vi "数据发送组合-20200825 (子VI).vi"(10 "枚举":T2(ring), 11 "插值后的数组元素":T1) -> (3 "字符串":string)   [LabVIEW 2016, in "数据传输系统-02.lvlib"]
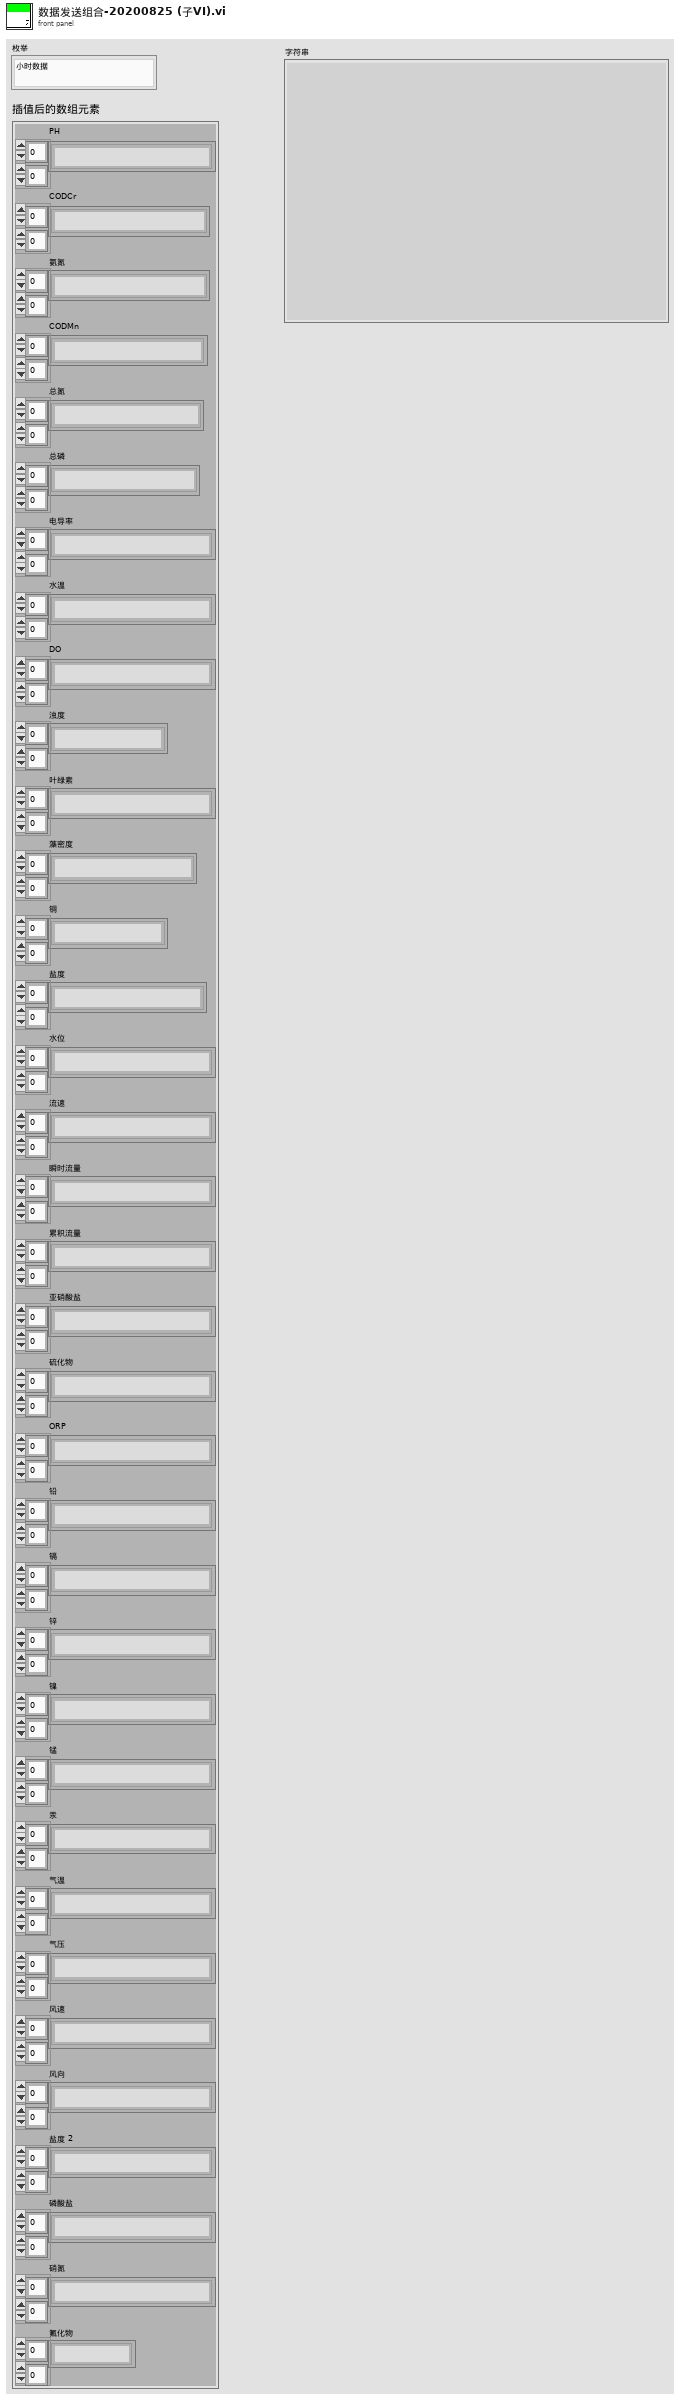
[diagram p1: front panel]
types:
  T1 = cluster{"PH":string[][], "CODCr":string[][], "氨氮":string[][], "CODMn":string[][], "总氮":string[][], "总磷":string[][], "电导率":string[][], "水温":string[][], "DO":string[][], "浊度":string[][], "叶绿素":string[][], "藻密度":string[][], "铜":string[][], "盐度":string[][], "水位":string[][], "流速":string[][], "瞬时流量":string[][], "累积流量":string[][], "亚硝酸盐":string[][], "硫化物":string[][], "ORP":string[][], "铅":string[][], "镉":string[][], "锌":string[][], "镍":string[][], "锰":string[][], "汞":string[][], "气温":string[][], "气压":string[][], "风速":string[][], "风向":string[][], "盐度 2":string[][], "磷酸盐":string[][], "硝氮":string[][], "氟化物":string[][]}
  T2 = enum16{"小时数据", "实时数据", "平行样测试", "集成干预测试", "加标回收测试", "核查数据", "空白零点跨度数据", "提取小时数据", "提取实时数据", "操作日志", "仪器参数", "3090仪器参数", "提取仪器参数", "报警信息"}
  T3 = cluster{"CODMn":dbl, "CODCr":dbl, "DO":dbl, "铜":dbl, "PH":dbl, "氨氮":dbl, "比电导率":dbl, "水温":dbl, "COD":dbl, "浊度":dbl, "总氮":dbl, "总磷":dbl, "叶绿素a":dbl, "藻密度":dbl, "水位":dbl, "流速":dbl, "瞬时流量":dbl, "累积流量":dbl, "亚硝酸盐":dbl, "硫化物":dbl, "ORP":dbl, "铅":dbl, "镉":dbl, "锌":dbl, "镍":dbl, "锰":dbl, "汞":dbl, "气温":dbl, "气压":dbl, "风速":dbl, "风向":dbl, "盐度":dbl, "磷酸盐":dbl, "硝氮":dbl, "氟化物":dbl}
  T4 = cluster{"CODMn":string, "CODCr":string, "DO":string, "铜":string, "PH":string, "氨氮":string, "比电导率":string, "水温":string, "COD":string, "浊度":string, "总氮":string, "总磷":string, "叶绿素a":string, "藻密度":string, "水位":string, "流速":string, "瞬时流量":string, "累积流量":string, "亚硝酸盐":string, "硫化物":string, "ORP":string, "铅":string, "镉":string, "锌":string, "镍":string, "锰":string, "汞":string, "气温":string, "气压":string, "风速":string, "风向":string, "盐度":string, "磷酸盐":string, "硝氮":string, "氟化物":string}
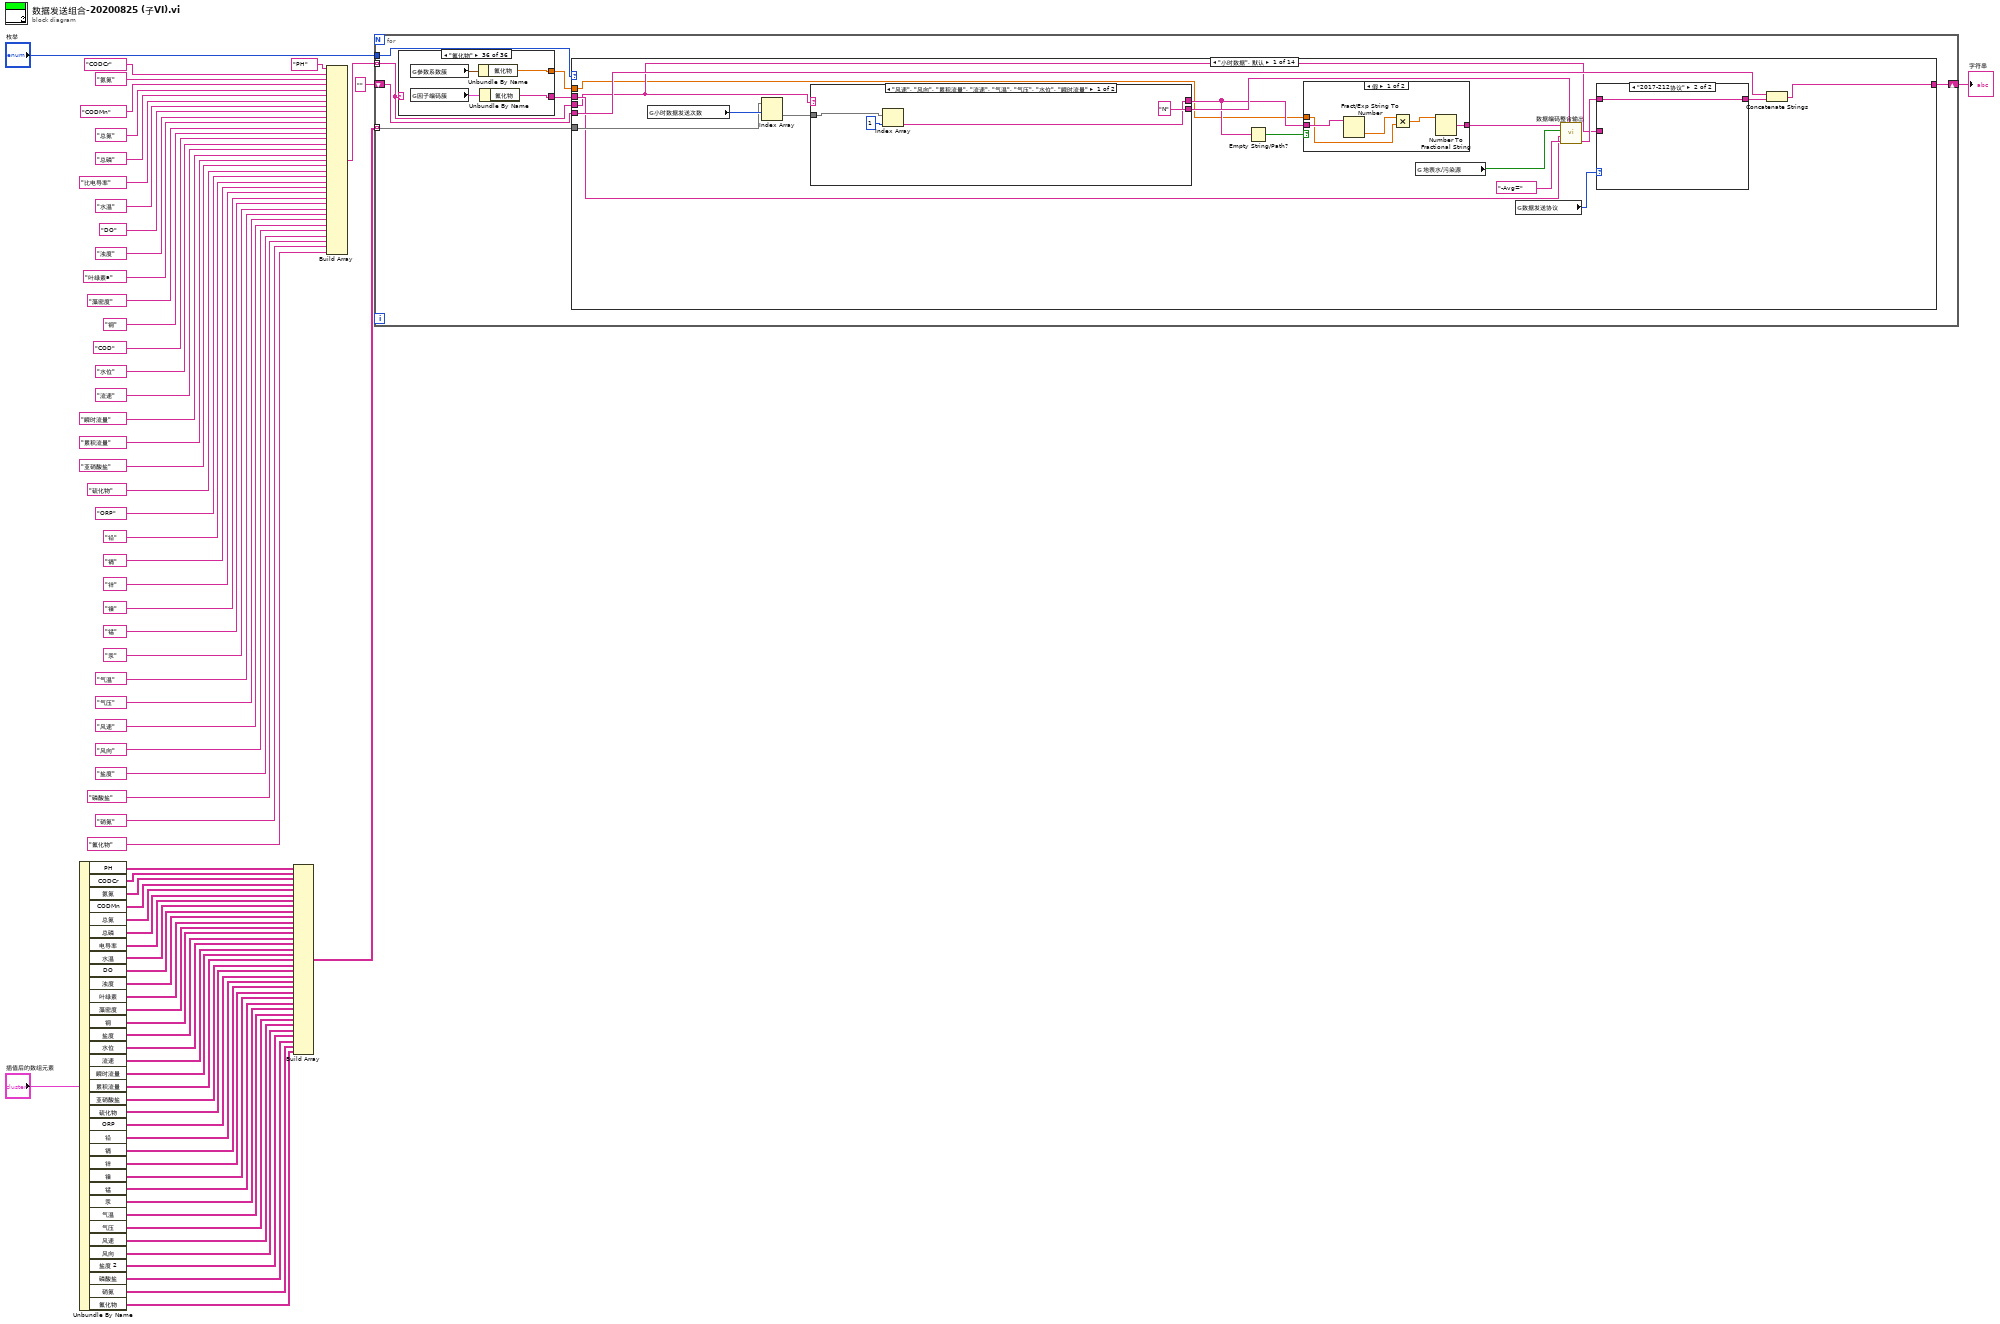
[diagram p0: block diagram]
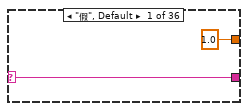
[diagram p2: hidden frame]
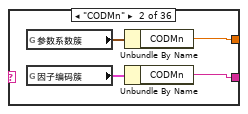
[diagram p3: hidden frame]
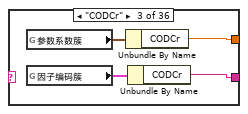
[diagram p4: hidden frame]
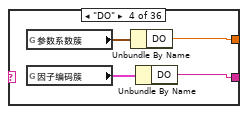
[diagram p5: hidden frame]
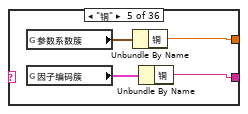
[diagram p6: hidden frame]
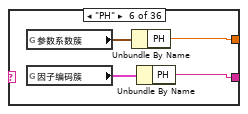
[diagram p7: hidden frame]
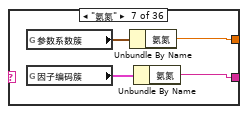
[diagram p8: hidden frame]
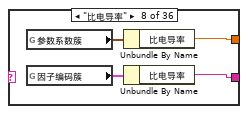
[diagram p9: hidden frame]
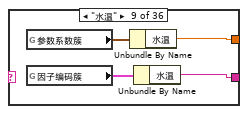
[diagram p10: hidden frame]
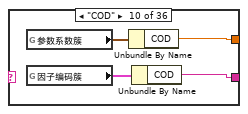
[diagram p11: hidden frame]
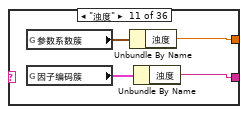
[diagram p12: hidden frame]
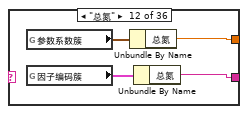
[diagram p13: hidden frame]
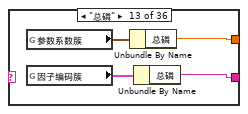
[diagram p14: hidden frame]
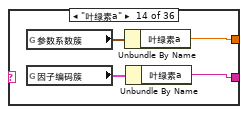
[diagram p15: hidden frame]
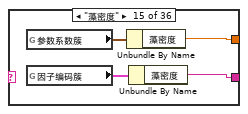
[diagram p16: hidden frame]
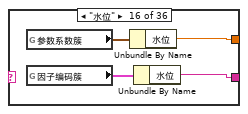
[diagram p17: hidden frame]
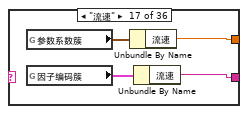
[diagram p18: hidden frame]
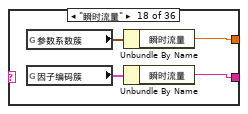
[diagram p19: hidden frame]
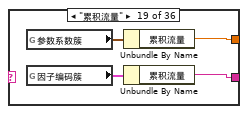
[diagram p20: hidden frame]
diagram:
  n1 = Unbundle By Name("插值后的数组元素") -> ("PH"=w76:string[][], "CODCr"=w75:string[][], "氨氮"=w74:string[][], "CODMn"=w73:string[][], "总氮"=w72:string[][], "总磷"=w71:string[][], "电导率"=w70:string[][], "水温"=w69:string[][], "DO"=w68:string[][], "浊度"=w67:string[][], "叶绿素"=w66:string[][], "藻密度"=w65:string[][], "铜"=w64:string[][], "盐度"=w63:string[][], "水位"=w62:string[][], "流速"=w61:string[][], "瞬时流量"=w60:string[][], "累积流量"=w59:string[][], "亚硝酸盐"=w58:string[][], "硫化物"=w57:string[][], "ORP"=w56:string[][], "铅"=w55:string[][], "镉"=w54:string[][], "锌"=w53:string[][], "镍"=w52:string[][], "锰"=w51:string[][], "汞"=w50:string[][], "气温"=w14:string[][], "气压"=w15:string[][], "风速"=w16:string[][], "风向"=w17:string[][], "盐度 2"=w8:string[][], "磷酸盐"=w7:string[][], "硝氮"=w6:string[][], "氟化物"=w2:string[][])
  n2 = Build Array(w76, w75, w74, w73, w72, w71, w70, w69, w68, w67, w66, w65, w64, w63, w62, w61, w60, w59, w58, w57, w56, w55, w54, w53, w52, w51, w50, w14, w15, w16, w17, w8, w7, w6, w2) -> (w49:string[][][])
  n3 = Build Array("PH" ("污染物编码"), "CODCr" ("污染物编码"), "氨氮" ("污染物编码"), "CODMn" ("污染物编码"), "总氮" ("污染物编码"), "总磷" ("污染物编码"), "比电导率" ("污染物编码"), "水温" ("污染物编码"), "DO" ("污染物编码"), "浊度" ("污染物编码"), "叶绿素a" ("污染物编码"), "藻密度" ("污染物编码"), "铜" ("污染物编码"), "COD" ("污染物编码"), "水位" ("污染物编码"), "流速" ("污染物编码"), "瞬时流量" ("污染物编码"), "累积流量" ("污染物编码"), "亚硝酸盐" ("污染物编码"), "硫化物" ("污染物编码"), "ORP" ("污染物编码"), "铅" ("污染物编码"), "镉" ("污染物编码"), "锌" ("污染物编码"), "镍" ("污染物编码"), "锰" ("污染物编码"), "汞" ("污染物编码"), "气温" ("污染物编码"), "气压" ("污染物编码"), "风速" ("污染物编码"), "风向" ("污染物编码"), "盐度" ("污染物编码"), "磷酸盐" ("污染物编码"), "硝氮" ("污染物编码"), "氟化物" ("污染物编码")) -> (w21:string[])
  n4 = for {
    tunnel: w49 -> [w83] mode=indexing
    tunnel: w21 -> [w78] mode=indexing
    shift-right: [w82] -> w19
    shift-left: "" -> [w81]
    tunnel: "枚举" -> [w80]
    n5 = case shown="\"氟化物\"" w78 {
      selector: w78 -> [w85 _ _ _ _ _ _ _ _ _ _ _ _ _ _ _ _ _ _ _ _ _ _ _ _ _ _ _ _ _ _ _ _ _ _ _]
      tunnel: [w85 w88 w92 w96 w100 w104 w108 w112 w116 w120 w124 w128 w132 w136 w140 w144 w148 w152 w156 w160 w164 w168 w172 w176 w180 w184 w188 w192 w196 w200 w204 w208 w212 w216 w220 w224] -> w79
      tunnel: [1.0 ("风向") w86 w90 w94 w98 w102 w106 w110 w114 w118 w122 w126 w130 w134 w138 w142 w146 w150 w154 w158 w162 w166 w170 w174 w178 w182 w186 w190 w194 w198 w202 w206 w210 w214 w218 w222] -> w77
      frame "假", Default {
      }
      frame "CODMn" {
        n6 = global read "断电保存全局.vi" "参数系数簇"() -> (w87:T3)
        n7 = global read "断电保存全局.vi" "因子编码簇"() -> (w89:T4)
        n8 = Unbundle By Name(w87) -> ("CODMn"=w86:dbl)
        n9 = Unbundle By Name(w89) -> ("CODMn"=w88:string)
      }
      frame "CODCr" {
        n10 = global read "断电保存全局.vi" "参数系数簇"() -> (w91:T3)
        n11 = global read "断电保存全局.vi" "因子编码簇"() -> (w93:T4)
        n12 = Unbundle By Name(w91) -> ("CODCr"=w90:dbl)
        n13 = Unbundle By Name(w93) -> ("CODCr"=w92:string)
      }
      frame "DO" {
        n14 = global read "断电保存全局.vi" "参数系数簇"() -> (w95:T3)
        n15 = global read "断电保存全局.vi" "因子编码簇"() -> (w97:T4)
        n16 = Unbundle By Name(w95) -> ("DO"=w94:dbl)
        n17 = Unbundle By Name(w97) -> ("DO"=w96:string)
      }
      frame "铜" {
        n18 = global read "断电保存全局.vi" "参数系数簇"() -> (w99:T3)
        n19 = global read "断电保存全局.vi" "因子编码簇"() -> (w101:T4)
        n20 = Unbundle By Name(w99) -> ("铜"=w98:dbl)
        n21 = Unbundle By Name(w101) -> ("铜"=w100:string)
      }
      frame "PH" {
        n22 = global read "断电保存全局.vi" "参数系数簇"() -> (w103:T3)
        n23 = global read "断电保存全局.vi" "因子编码簇"() -> (w105:T4)
        n24 = Unbundle By Name(w103) -> ("PH"=w102:dbl)
        n25 = Unbundle By Name(w105) -> ("PH"=w104:string)
      }
      frame "氨氮" {
        n26 = global read "断电保存全局.vi" "参数系数簇"() -> (w107:T3)
        n27 = global read "断电保存全局.vi" "因子编码簇"() -> (w109:T4)
        n28 = Unbundle By Name(w107) -> ("氨氮"=w106:dbl)
        n29 = Unbundle By Name(w109) -> ("氨氮"=w108:string)
      }
      frame "比电导率" {
        n30 = global read "断电保存全局.vi" "参数系数簇"() -> (w111:T3)
        n31 = global read "断电保存全局.vi" "因子编码簇"() -> (w113:T4)
        n32 = Unbundle By Name(w111) -> ("比电导率"=w110:dbl)
        n33 = Unbundle By Name(w113) -> ("比电导率"=w112:string)
      }
      frame "水温" {
        n34 = global read "断电保存全局.vi" "参数系数簇"() -> (w115:T3)
        n35 = global read "断电保存全局.vi" "因子编码簇"() -> (w117:T4)
        n36 = Unbundle By Name(w115) -> ("水温"=w114:dbl)
        n37 = Unbundle By Name(w117) -> ("水温"=w116:string)
      }
      frame "COD" {
        n38 = global read "断电保存全局.vi" "参数系数簇"() -> (w119:T3)
        n39 = global read "断电保存全局.vi" "因子编码簇"() -> (w121:T4)
        n40 = Unbundle By Name(w119) -> ("COD"=w118:dbl)
        n41 = Unbundle By Name(w121) -> ("COD"=w120:string)
      }
      frame "浊度" {
        n42 = global read "断电保存全局.vi" "参数系数簇"() -> (w123:T3)
        n43 = global read "断电保存全局.vi" "因子编码簇"() -> (w125:T4)
        n44 = Unbundle By Name(w123) -> ("浊度"=w122:dbl)
        n45 = Unbundle By Name(w125) -> ("浊度"=w124:string)
      }
      frame "总氮" {
        n46 = global read "断电保存全局.vi" "参数系数簇"() -> (w127:T3)
        n47 = global read "断电保存全局.vi" "因子编码簇"() -> (w129:T4)
        n48 = Unbundle By Name(w127) -> ("总氮"=w126:dbl)
        n49 = Unbundle By Name(w129) -> ("总氮"=w128:string)
      }
      frame "总磷" {
        n50 = global read "断电保存全局.vi" "参数系数簇"() -> (w131:T3)
        n51 = global read "断电保存全局.vi" "因子编码簇"() -> (w133:T4)
        n52 = Unbundle By Name(w131) -> ("总磷"=w130:dbl)
        n53 = Unbundle By Name(w133) -> ("总磷"=w132:string)
      }
      frame "叶绿素a" {
        n54 = global read "断电保存全局.vi" "参数系数簇"() -> (w135:T3)
        n55 = global read "断电保存全局.vi" "因子编码簇"() -> (w137:T4)
        n56 = Unbundle By Name(w135) -> ("叶绿素a"=w134:dbl)
        n57 = Unbundle By Name(w137) -> ("叶绿素a"=w136:string)
      }
      frame "藻密度" {
        n58 = global read "断电保存全局.vi" "参数系数簇"() -> (w139:T3)
        n59 = global read "断电保存全局.vi" "因子编码簇"() -> (w141:T4)
        n60 = Unbundle By Name(w139) -> ("藻密度"=w138:dbl)
        n61 = Unbundle By Name(w141) -> ("藻密度"=w140:string)
      }
      frame "水位" {
        n62 = global read "断电保存全局.vi" "参数系数簇"() -> (w143:T3)
        n63 = global read "断电保存全局.vi" "因子编码簇"() -> (w145:T4)
        n64 = Unbundle By Name(w143) -> ("水位"=w142:dbl)
        n65 = Unbundle By Name(w145) -> ("水位"=w144:string)
      }
      frame "流速" {
        n66 = global read "断电保存全局.vi" "参数系数簇"() -> (w147:T3)
        n67 = global read "断电保存全局.vi" "因子编码簇"() -> (w149:T4)
        n68 = Unbundle By Name(w147) -> ("流速"=w146:dbl)
        n69 = Unbundle By Name(w149) -> ("流速"=w148:string)
      }
      frame "瞬时流量" {
        n70 = global read "断电保存全局.vi" "参数系数簇"() -> (w151:T3)
        n71 = global read "断电保存全局.vi" "因子编码簇"() -> (w153:T4)
        n72 = Unbundle By Name(w151) -> ("瞬时流量"=w150:dbl)
        n73 = Unbundle By Name(w153) -> ("瞬时流量"=w152:string)
      }
      frame "累积流量" {
        n74 = global read "断电保存全局.vi" "参数系数簇"() -> (w155:T3)
        n75 = global read "断电保存全局.vi" "因子编码簇"() -> (w157:T4)
        n76 = Unbundle By Name(w155) -> ("累积流量"=w154:dbl)
        n77 = Unbundle By Name(w157) -> ("累积流量"=w156:string)
      }
      frame "亚硝酸盐" {
        n78 = global read "断电保存全局.vi" "参数系数簇"() -> (w159:T3)
        n79 = global read "断电保存全局.vi" "因子编码簇"() -> (w161:T4)
        n80 = Unbundle By Name(w159) -> ("亚硝酸盐"=w158:dbl)
        n81 = Unbundle By Name(w161) -> ("亚硝酸盐"=w160:string)
      }
      frame "硫化物" {
        n82 = global read "断电保存全局.vi" "参数系数簇"() -> (w163:T3)
        n83 = global read "断电保存全局.vi" "因子编码簇"() -> (w165:T4)
        n84 = Unbundle By Name(w163) -> ("硫化物"=w162:dbl)
        n85 = Unbundle By Name(w165) -> ("硫化物"=w164:string)
      }
      frame "ORP" {
        n86 = global read "断电保存全局.vi" "参数系数簇"() -> (w167:T3)
        n87 = global read "断电保存全局.vi" "因子编码簇"() -> (w169:T4)
        n88 = Unbundle By Name(w167) -> ("ORP"=w166:dbl)
        n89 = Unbundle By Name(w169) -> ("ORP"=w168:string)
      }
      frame "铅" {
        n90 = global read "断电保存全局.vi" "参数系数簇"() -> (w171:T3)
        n91 = global read "断电保存全局.vi" "因子编码簇"() -> (w173:T4)
        n92 = Unbundle By Name(w171) -> ("铅"=w170:dbl)
        n93 = Unbundle By Name(w173) -> ("铅"=w172:string)
      }
      frame "镉" {
        n94 = global read "断电保存全局.vi" "参数系数簇"() -> (w175:T3)
        n95 = global read "断电保存全局.vi" "因子编码簇"() -> (w177:T4)
        n96 = Unbundle By Name(w175) -> ("镉"=w174:dbl)
        n97 = Unbundle By Name(w177) -> ("镉"=w176:string)
      }
      frame "锌" {
        n98 = global read "断电保存全局.vi" "参数系数簇"() -> (w179:T3)
        n99 = global read "断电保存全局.vi" "因子编码簇"() -> (w181:T4)
        n100 = Unbundle By Name(w179) -> ("锌"=w178:dbl)
        n101 = Unbundle By Name(w181) -> ("锌"=w180:string)
      }
      frame "镍" {
        n102 = global read "断电保存全局.vi" "参数系数簇"() -> (w183:T3)
        n103 = global read "断电保存全局.vi" "因子编码簇"() -> (w185:T4)
        n104 = Unbundle By Name(w183) -> ("镍"=w182:dbl)
        n105 = Unbundle By Name(w185) -> ("镍"=w184:string)
      }
      frame "锰" {
        n106 = global read "断电保存全局.vi" "参数系数簇"() -> (w187:T3)
        n107 = global read "断电保存全局.vi" "因子编码簇"() -> (w189:T4)
        n108 = Unbundle By Name(w187) -> ("锰"=w186:dbl)
        n109 = Unbundle By Name(w189) -> ("锰"=w188:string)
      }
      frame "汞" {
        n110 = global read "断电保存全局.vi" "参数系数簇"() -> (w191:T3)
        n111 = global read "断电保存全局.vi" "因子编码簇"() -> (w193:T4)
        n112 = Unbundle By Name(w191) -> ("汞"=w190:dbl)
        n113 = Unbundle By Name(w193) -> ("汞"=w192:string)
      }
      frame "气温" {
        n114 = global read "断电保存全局.vi" "参数系数簇"() -> (w195:T3)
        n115 = global read "断电保存全局.vi" "因子编码簇"() -> (w197:T4)
        n116 = Unbundle By Name(w195) -> ("气温"=w194:dbl)
        n117 = Unbundle By Name(w197) -> ("气温"=w196:string)
      }
      frame "气压" {
        n118 = global read "断电保存全局.vi" "参数系数簇"() -> (w199:T3)
        n119 = global read "断电保存全局.vi" "因子编码簇"() -> (w201:T4)
        n120 = Unbundle By Name(w199) -> ("气压"=w198:dbl)
        n121 = Unbundle By Name(w201) -> ("气压"=w200:string)
      }
      frame "风速" {
        n122 = global read "断电保存全局.vi" "参数系数簇"() -> (w203:T3)
        n123 = global read "断电保存全局.vi" "因子编码簇"() -> (w205:T4)
        n124 = Unbundle By Name(w203) -> ("风速"=w202:dbl)
        n125 = Unbundle By Name(w205) -> ("风速"=w204:string)
      }
      frame "风向" {
        n126 = global read "断电保存全局.vi" "参数系数簇"() -> (w207:T3)
        n127 = global read "断电保存全局.vi" "因子编码簇"() -> (w209:T4)
        n128 = Unbundle By Name(w207) -> ("风向"=w206:dbl)
        n129 = Unbundle By Name(w209) -> ("风向"=w208:string)
      }
      frame "盐度" {
        n130 = global read "断电保存全局.vi" "参数系数簇"() -> (w211:T3)
        n131 = global read "断电保存全局.vi" "因子编码簇"() -> (w213:T4)
        n132 = Unbundle By Name(w211) -> ("盐度"=w210:dbl)
        n133 = Unbundle By Name(w213) -> ("盐度"=w212:string)
      }
      frame "磷酸盐" {
        n134 = global read "断电保存全局.vi" "参数系数簇"() -> (w215:T3)
        n135 = global read "断电保存全局.vi" "因子编码簇"() -> (w217:T4)
        n136 = Unbundle By Name(w215) -> ("磷酸盐"=w214:dbl)
        n137 = Unbundle By Name(w217) -> ("磷酸盐"=w216:string)
      }
      frame "硝氮" {
        n138 = global read "断电保存全局.vi" "参数系数簇"() -> (w219:T3)
        n139 = global read "断电保存全局.vi" "因子编码簇"() -> (w221:T4)
        n140 = Unbundle By Name(w219) -> ("硝氮"=w218:dbl)
        n141 = Unbundle By Name(w221) -> ("硝氮"=w220:string)
      }
      frame "氟化物" {
        n142 = global read "断电保存全局.vi" "参数系数簇"() -> (w223:T3)
        n143 = global read "断电保存全局.vi" "因子编码簇"() -> (w225:T4)
        n144 = Unbundle By Name(w223) -> ("氟化物"=w222:dbl)
        n145 = Unbundle By Name(w225) -> ("氟化物"=w224:string)
      }
    }
    n146 = case shown="\"小时数据\", 默认" w80 {
      tunnel: w83 -> [w238 w282 w313 w322 w376 w383 w393 w417 w439 w476 w494 w501 w511 w533]
      tunnel: w79 -> [w234 w275 w312 w323 w377 w382 w392 w411 w438 w464 w492 w499 w510 w536]
      tunnel: [w237 w279 w314 w320 w378 w379 w389 w408 w437 w471 w489 w498 w506 w521] -> w82
      tunnel: w81 -> [w236 w280 w316 w321 w373 w381 w390 w409 w440 w472 w490 w500 w507 w516]
      tunnel: w78 -> [w231 w274 _ w317 _ _ _ _ _ _ _ _ _ w531]
      tunnel: w77 -> [w228 w270 _ w318 _ _ _ w404 w433 _ _ _ _ _]
      frame "小时数据", Default {
        n147 = global read "全局 小时数据发送次数.vi" "小时数据发送次数"() -> (w242:i32)
        n148 = Index Array(array=w238, index (row)=w242) -> (element=w241:string[])  [unwired: 1 in]
        n149 = case shown="\"风速\", \"风向\", \"累积流量\", \"流速\", \"气温\", \"气压\", \"水位\", \"瞬时流量\"" w231 {
          tunnel: w241 -> [w252 w255]
          tunnel: [w249 w254] -> w229
          tunnel: ["N" ("字符串") w253] -> w239
          frame "风速", "风向", "累积流量", "流速", "气温", "气压", "水位", "瞬时流量" {
            n150 = Index Array(array=w252, index=1 ("索引")) -> (element=w249:string)
          }
          frame "", Default {
            n151 = Index Array(array=w255, index #1=2 ("索引"), index #2=3 ("索引"), index #3=5 ("索引")) -> (element #1=w258:string, element #2=w257:string, element #3=w253:string)
            n152 = case shown="\"N\", 默认" w258 {
              tunnel: [w261 ""] -> w254
              tunnel: w257 -> [w261 _]
              frame "N", Default {
              }
              frame "M" {
              }
            }
          }
        }
        n153 = Empty String/Path?(string/path=w229) -> (empty?=w230:bool)
        n154 = case shown="假" w230 {
          tunnel: w229 -> [w246 w248]
          tunnel: w228 -> [w245 _]
          tunnel: [w243 w248] -> w227
          frame False {
            n155 = Fract/Exp String To Number(string=w246) -> (number=w247:dbl)  [unwired: 3 in, 1 out]
            n156 = Multiply(x=w247, y=w245) -> (x*y=w244:dbl)
            n157 = Number To Fractional String(number=w244) -> (F-format string=w243:string)  [unwired: 3 in]
          }
          frame True {
            # "空"
          }
        }
        n158 = global read "断电保存全局.vi" "地表水/污染源"() -> (w226:bool)
        n159 = global read "断电保存全局.vi" "数据发送协议"() -> (w235:enum16{"2005-212协议", "2017-212协议"})
        n160 = call "数据编码整合输出.vi"("数据标识"=w239, "数据类型"="-Avg=", "污染物编码"=w234, "地表水/污染源"=w226, "数据值"=w227) -> ("编码输出"=w233:string)  [unwired: 6 in]
        n161 = case shown="\"2017-212协议\"" w235 {
          tunnel: w231 -> [w265 _]
          tunnel: w233 -> [w263 w268]
          tunnel: [w264 w268] -> w232
          frame "2005-212协议", Default {
            n162 = case shown="\"风速\", \"风向\", \"累积流量\", \"流速\", \"气温\", \"气压\", \"水位\"" w265 {
              tunnel: [w266 ""] -> w264
              tunnel: w263 -> [w266 _]
              frame "假", Default {
              }
              frame "风速", "风向", "累积流量", "流速", "气温", "气压", "水位" {
              }
            }
          }
          frame "2017-212协议" {
          }
        }
        n163 = Concatenate Strings(w236, w232) -> (w237:string)
      }
      frame "实时数据" {
        n164 = global read "全局 小时数据发送次数.vi" "小时数据发送次数"() -> (w283:i32)
        n165 = Index Array(array=w282, index (row)=w283) -> (element=w284:string[])  [unwired: 1 in]
        n166 = case shown="\"\", 默认" w274 {
          tunnel: w284 -> [w293 w297 w303]
          tunnel: [w292 w296 w302] -> w272
          tunnel: ["N" ("字符串") "N" ("字符串") w300] -> w281
          frame "累积流量", "流速", "水位", "瞬时流量" {
            n167 = Index Array(array=w293, index=1 ("索引")) -> (element=w292:string)
          }
          frame "风速", "风向", "气温", "气压" {
            n168 = Index Array(array=w297, index=1 ("索引")) -> (element=w296:string)
          }
          frame "", Default {
            n169 = Index Array(array=w303, index #1=3 ("索引"), index #2=5 ("索引")) -> (element #1=w302:string, element #2=w300:string)
          }
        }
        n170 = Empty String/Path?(string/path=w272) -> (empty?=w273:bool)
        n171 = case shown="假" w273 {
          tunnel: w272 -> [w289 w291]
          tunnel: w270 -> [w288 _]
          tunnel: [w286 w291] -> w271
          frame False {
            n172 = Fract/Exp String To Number(string=w289) -> (number=w290:dbl)  [unwired: 3 in, 1 out]
            n173 = Multiply(x=w290, y=w288) -> (x*y=w287:dbl)
            n174 = Number To Fractional String(number=w287) -> (F-format string=w286:string)  [unwired: 3 in]
          }
          frame True {
            # "空"
          }
        }
        n175 = global read "断电保存全局.vi" "数据发送协议"() -> (w278:enum16{"2005-212协议", "2017-212协议"})
        n176 = call "数据编码整合输出.vi"("数据标识"=w281, "数据类型"="-Rtd=", "污染物编码"=w275, "地表水/污染源"=FALSE, "数据值"=w271) -> ("编码输出"=w277:string)  [unwired: 6 in]
        n177 = case shown="\"2017-212协议\"" w278 {
          tunnel: w274 -> [w307 _]
          tunnel: w277 -> [w305 w310]
          tunnel: [w306 w310] -> w276
          frame "2005-212协议", Default {
            n178 = case shown="\"假\", 默认" w307 {
              tunnel: [w308 ""] -> w306
              tunnel: w305 -> [w308 _]
              frame "假", Default {
              }
              frame "风速", "风向", "累积流量", "流速", "气温", "气压", "水位" {
              }
            }
          }
          frame "2017-212协议" {
          }
        }
        n179 = Concatenate Strings(w280, w276) -> (w279:string)
      }
      frame "平行样测试" {
        n180 = global read "全局 小时数据发送次数.vi" "小时数据发送次数"() -> (w311:i32)
        n181 = call "平行样集成干预数据组合(子VI).vi"("污染物编码"=w312, "数据输入"=w313, "小时数据发送次数"=w311) -> ("输出组合"=w315:string)  [unwired: 8 in]
        n182 = Concatenate Strings(w316, w315) -> (w314:string)
      }
      frame "集成干预测试" {
        n183 = global read "断电保存全局.vi" "应用环境"() -> (w319:enum16{"STD", "GB212"})
        n184 = case shown="\"GB212\"" w319 {
          tunnel: w323 -> [w327 w333]
          tunnel: w322 -> [w326 w334]
          tunnel: w321 -> [w325 w335]
          tunnel: [w324 w330] -> w320
          tunnel: w318 -> [_ w332]
          tunnel: w317 -> [_ w331]
          frame "STD", Default {
            n185 = global read "全局 小时数据发送次数.vi" "小时数据发送次数"() -> (w328:i32)
            n186 = call "平行样集成干预数据组合(子VI).vi"("污染物编码"=w327, "数据输入"=w326, "小时数据发送次数"=w328) -> ("输出组合"=w329:string)  [unwired: 8 in]
            n187 = Concatenate Strings(w325, w329) -> (w324:string)
          }
          frame "GB212" {
            n188 = global read "全局 小时数据发送次数.vi" "小时数据发送次数"() -> (w346:i32)
            n189 = Index Array(array=w334, index (row)=w346) -> (element=w345:string[])  [unwired: 1 in]
            n190 = case shown="\"\", 默认" w331 {
              tunnel: w345 -> [w356 w359]
              tunnel: [w353 w358] -> w338
              tunnel: ["N" ("字符串") w357] -> w343
              frame "风速", "风向", "累积流量", "流速", "气温", "气压", "水位", "瞬时流量" {
                n191 = Index Array(array=w356, index=1 ("索引")) -> (element=w353:string)
              }
              frame "", Default {
                n192 = Index Array(array=w359, index #1=2 ("索引"), index #2=3 ("索引"), index #3=5 ("索引")) -> (element #1=w362:string, element #2=w361:string, element #3=w357:string)
                n193 = case shown="\"N\", 默认" w362 {
                  tunnel: [w365 ""] -> w358
                  tunnel: w361 -> [w365 _]
                  frame "N", Default {
                  }
                  frame "M" {
                  }
                }
              }
            }
            n194 = Empty String/Path?(string/path=w338) -> (empty?=w339:bool)
            n195 = case shown="假" w339 {
              tunnel: w338 -> [w350 w352]
              tunnel: w332 -> [w349 _]
              tunnel: [w347 w352] -> w337
              frame False {
                n196 = Fract/Exp String To Number(string=w350) -> (number=w351:dbl)  [unwired: 3 in, 1 out]
                n197 = Multiply(x=w351, y=w349) -> (x*y=w348:dbl)
                n198 = Number To Fractional String(number=w348) -> (F-format string=w347:string)  [unwired: 3 in]
              }
              frame True {
                # "空"
              }
            }
            n199 = global read "断电保存全局.vi" "地表水/污染源"() -> (w336:bool)
            n200 = global read "断电保存全局.vi" "数据发送协议"() -> (w342:enum16{"2005-212协议", "2017-212协议"})
            n201 = call "数据编码整合输出.vi"("数据标识"=w343, "数据类型"="-Avg=", "污染物编码"=w333, "地表水/污染源"=w336, "数据值"=w337) -> ("编码输出"=w341:string)  [unwired: 6 in]
            n202 = case shown="\"2017-212协议\"" w342 {
              tunnel: w331 -> [w369 _]
              tunnel: w341 -> [w367 w372]
              tunnel: [w368 w372] -> w340
              frame "2005-212协议", Default {
                n203 = case shown="\"假\", 默认" w369 {
                  tunnel: [w370 ""] -> w368
                  tunnel: w367 -> [w370 _]
                  frame "假", Default {
                  }
                  frame "风速", "风向", "累积流量", "流速", "气温", "气压", "水位" {
                  }
                }
              }
              frame "2017-212协议" {
              }
            }
            n204 = Concatenate Strings(w335, w340) -> (w330:string)
          }
        }
      }
      frame "加标回收测试" {
        n205 = global read "全局 小时数据发送次数.vi" "小时数据发送次数"() -> (w375:i32)
        n206 = call "加标回收数据组合 (子VI).vi"("小时数据发送次数"=w375, "数据"=w376, "污染物编码"=w377) -> ("组合输出"=w374:string)  [unwired: 7 in, 1 out]
        n207 = Concatenate Strings(w373, w374) -> (w378:string)
      }
      frame "核查数据" {
        n208 = global read "全局 小时数据发送次数.vi" "小时数据发送次数"() -> (w384:i32)
        n209 = call "标样核查数据组合(子VI).vi"("小时数据发送次数"=w384, "数据输入"=w383, "污染物编码"=w382) -> ("输出组合"=w380:string)  [unwired: 8 in]
        n210 = Concatenate Strings(w381, w380) -> (w379:string)
      }
      frame "空白零点跨度数据" {
        n211 = global read "全局 小时数据发送次数.vi" "小时数据发送次数"() -> (w395:i32)
        n212 = Index Array(array=w393, index (row)=w395) -> (element=w399:string[])  [unwired: 1 in]
        n213 = Index Array(array=w399, index #1=0 ("索引"), index #2=3 ("索引"), index #3=6 ("索引"), index #4=7 ("索引")) -> (element #2=w394:string, element #3=w396:string, element #4=w385:string)  [unwired: 1 out]
        n214 = Empty String/Path?(string/path=w385) -> (empty?=w387:bool)
        n215 = case shown="假" w387 {
          tunnel: [w401 "0" ("span value")] -> w386
          tunnel: w385 -> [w401 _]
          frame False {
          }
          frame True {
          }
        }
        n216 = call "零点跨度数据组合 (子VI).vi"("span value"=w386, "standard value"=w396, "check value"=w394, "污染物编码"=w392) -> ("组合输出"=w391:string)  [unwired: 7 in]
        n217 = Concatenate Strings(w390, w391) -> (w389:string)
      }
      frame "提取小时数据" {
        n218 = global read "全局 小时数据发送次数.vi" "小时数据发送次数"() -> (w418:i32)
        n219 = Index Array(array=w417, index (row)=w418) -> (element=w416:string[])  [unwired: 1 in]
        n220 = Index Array(array=w416, index #2=1 ("索引")) -> (element #2=w405:string)  [unwired: 1 in, 1 out]
        n221 = Empty String/Path?(string/path=w405) -> (empty?=w407:bool)
        n222 = case shown="假" w407 {
          tunnel: w405 -> [w423 w425]
          tunnel: w404 -> [w422 _]
          tunnel: [w420 w425] -> w406
          frame False {
            n223 = Fract/Exp String To Number(string=w423) -> (number=w424:dbl)  [unwired: 3 in, 1 out]
            n224 = Multiply(x=w424, y=w422) -> (x*y=w421:dbl)
            n225 = Number To Fractional String(number=w421) -> (F-format string=w420:string)  [unwired: 3 in]
          }
          frame True {
            # "空"
          }
        }
        n226 = global read "断电保存全局.vi" "地表水/污染源"() -> (w403:bool)
        n227 = global read "断电保存全局.vi" "数据发送协议"() -> (w413:enum16{"2005-212协议", "2017-212协议"})
        n228 = call "数据编码整合输出.vi"("数据标识"="N", "数据类型"="-Avg=", "污染物编码"=w411, "地表水/污染源"=w403, "数据值"=w406) -> ("编码输出"=w410:string)  [unwired: 6 in]
        n229 = case shown="\"2005-212协议\", 默认" w413 {
          tunnel: w411 -> [w428 _]
          tunnel: w410 -> [w426 w431]
          tunnel: [w427 w431] -> w412
          frame "2005-212协议", Default {
            n230 = case shown="\"假\", 默认" w428 {
              tunnel: [w429 ""] -> w427
              tunnel: w426 -> [w429 _]
              frame "假", Default {
              }
              frame "累积流量", "流速", "水位" {
              }
            }
          }
          frame "2017-212协议" {
          }
        }
        n231 = Concatenate Strings(w409, w412) -> (w408:string)
      }
      frame "提取实时数据" {
        n232 = global read "全局 小时数据发送次数.vi" "小时数据发送次数"() -> (w446:i32)
        n233 = Index Array(array=w439, index (row)=w446) -> (element=w447:string[])  [unwired: 1 in]
        n234 = Index Array(array=w447, index #1=3 ("索引"), index #2=5 ("索引")) -> (element #1=w434:string, element #2=w444:string)
        n235 = Empty String/Path?(string/path=w434) -> (empty?=w436:bool)
        n236 = case shown="假" w436 {
          tunnel: w434 -> [w453 w455]
          tunnel: w433 -> [w452 _]
          tunnel: [w450 w455] -> w435
          frame False {
            n237 = Fract/Exp String To Number(string=w453) -> (number=w454:dbl)  [unwired: 3 in, 1 out]
            n238 = Multiply(x=w454, y=w452) -> (x*y=w451:dbl)
            n239 = Number To Fractional String(number=w451) -> (F-format string=w450:string)  [unwired: 3 in]
          }
          frame True {
            # "空"
          }
        }
        n240 = global read "断电保存全局.vi" "地表水/污染源"() -> (w432:bool)
        n241 = global read "断电保存全局.vi" "数据发送协议"() -> (w443:enum16{"2005-212协议", "2017-212协议"})
        n242 = call "数据编码整合输出.vi"("数据标识"=w444, "数据类型"="-Rtd=", "污染物编码"=w438, "地表水/污染源"=w432, "数据值"=w435) -> ("编码输出"=w442:string)  [unwired: 6 in]
        n243 = case shown="\"2017-212协议\"" w443 {
          tunnel: w438 -> [w458 _]
          tunnel: w442 -> [w456 w461]
          tunnel: [w457 w461] -> w441
          frame "2005-212协议", Default {
            n244 = case shown="\"累积流量\", \"流速\", \"水位\"" w458 {
              tunnel: [w459 ""] -> w457
              tunnel: w456 -> [w459 _]
              frame "假", Default {
              }
              frame "累积流量", "流速", "水位" {
              }
            }
          }
          frame "2017-212协议" {
          }
        }
        n245 = Concatenate Strings(w440, w441) -> (w437:string)
      }
      frame "操作日志" {
        n246 = global read "断电保存全局.vi" "因子编码簇"() -> (w467:T4)
        n247 = global read "全局 小时数据发送次数.vi" "小时数据发送次数"() -> (w480:i32)
        n248 = Unbundle By Name(w467) -> ("DO"=w466:string)
        n249 = Equal?(x=w464, y=w466) -> (x = y?=w462:bool)
        n250 = Index Array(array=w476, index (row)=w480) -> (element=w475:string[])  [unwired: 1 in]
        n251 = Index Array(array=w475, index #1=0 ("索引"), index #2=2 ("索引")) -> (element #2=w474:string)  [unwired: 1 out]
        n252 = Empty String/Path?(string/path=w474) -> (empty?=w479:bool)
        n253 = Select(t="w00000", s=w462, f=w464) -> (s? t:f=w463:string)
        n254 = Select(t="i21001", s=w462, f="i11001") -> (s? t:f=w468:string)
        n255 = case shown="假" w479 {
          tunnel: [w484 ""] -> w473
          tunnel: w474 -> [w482 _]
          tunnel: w463 -> [w483 _]
          tunnel: w468 -> [w481 _]
          frame False {
            n256 = Format Into String(format string="PolId=%s,%s-Info=//%s//;" ("格式字符串"), w483, w481, w482) -> (resulting string=w484:string)  [unwired: 2 in, 1 out]
          }
          frame True {
          }
        }
        n257 = Concatenate Strings(w472, w473) -> (w471:string)
      }
      frame "仪器参数" {
        n258 = global read "断电保存全局.vi" "应用环境"() -> (w488:enum16{"STD", "GB212"})
        n259 = global read "全局 小时数据发送次数.vi" "小时数据发送次数"() -> (w495:i32)
        n260 = case shown="\"STD\", 默认" w488 {
          tunnel: ["3090仪器参数" ("table") "仪器参数" ("table")] -> w487
          frame "STD", Default {
          }
          frame "GB212" {
          }
        }
        n261 = Index Array(array=w494, index (row)=w495) -> (element=w493:string[])  [unwired: 1 in]
        n262 = call "关键参数组合 (子VI).vi"("table"=w487, "因子编码"=w492, "data"=w493) -> ("字符串"=w491:string)  [unwired: 8 in]
        n263 = Concatenate Strings(w490, w491) -> (w489:string)
      }
      frame "3090仪器参数" {
        n264 = global read "全局 小时数据发送次数.vi" "小时数据发送次数"() -> (w505:i32)
        n265 = Index Array(array=w501, index (row)=w505) -> (element=w503:string[])  [unwired: 1 in]
        n266 = call "关键参数组合 (子VI).vi"("table"="3090仪器参数", "因子编码"=w499, "data"=w503) -> ("字符串"=w502:string)  [unwired: 8 in]
        n267 = Concatenate Strings(w500, w502) -> (w498:string)
      }
      frame "提取仪器参数" {
        n268 = global read "全局 小时数据发送次数.vi" "小时数据发送次数"() -> (w512:i32)
        n269 = Index Array(array=w511, index (row)=w512) -> (element=w509:string[])  [unwired: 1 in]
        n270 = call "提取仪器参数 (子VI).vi"("因子编码"=w510, "数据输入"=w509) -> ("字符串"=w508:string)  [unwired: 9 in]
        n271 = Concatenate Strings(w507, w508) -> (w506:string)
      }
      frame "报警信息" {
        n272 = Empty String/Path?(string/path=w516) -> (empty?=w515:bool)
        n273 = global read "断电保存全局.vi" "因子编码簇"() -> (w539:T4)
        n274 = case shown="\"CODMn\"" w531 {
          tunnel: [u16 0 ("register") w557 w563 w569 w575 w581] -> w529
          tunnel: [u16 0 ("register") w554 w560 w566 w572 w578] -> w513
          frame "假", Default {
          }
          frame "CODMn" {
            n275 = global read "全局1.vi" "读取试剂余量的值"() -> (w555:u16[])
            n276 = global read "全局1.vi" "register values"() -> (w559:u16[])
            n277 = Index Array(array=w559, index=1 ("索引")) -> (element=w557:u16)
            n278 = Index Array(array=w555, index=1 ("索引")) -> (element=w554:u16)
          }
          frame "氨氮" {
            n279 = global read "全局1.vi" "读取试剂余量的值"() -> (w561:u16[])
            n280 = global read "全局1.vi" "register values"() -> (w565:u16[])
            n281 = Index Array(array=w565, index=2 ("索引")) -> (element=w563:u16)
            n282 = Index Array(array=w561, index=2 ("索引")) -> (element=w560:u16)
          }
          frame "总磷" {
            n283 = global read "全局1.vi" "读取试剂余量的值"() -> (w567:u16[])
            n284 = global read "全局1.vi" "register values"() -> (w571:u16[])
            n285 = Index Array(array=w571, index=3 ("索引")) -> (element=w569:u16)
            n286 = Index Array(array=w567, index=3 ("索引")) -> (element=w566:u16)
          }
          frame "总氮" {
            n287 = global read "全局1.vi" "读取试剂余量的值"() -> (w573:u16[])
            n288 = global read "全局1.vi" "register values"() -> (w577:u16[])
            n289 = Index Array(array=w577, index=4 ("索引")) -> (element=w575:u16)
            n290 = Index Array(array=w573, index=4 ("索引")) -> (element=w572:u16)
          }
          frame "CODCr" {
            n291 = global read "全局1.vi" "读取试剂余量的值"() -> (w579:u16[])
            n292 = global read "全局1.vi" "register values"() -> (w583:u16[])
            n293 = Index Array(array=w583, index=5 ("索引")) -> (element=w581:u16)
            n294 = Index Array(array=w579, index=5 ("索引")) -> (element=w578:u16)
          }
        }
        n295 = global read "全局 小时数据发送次数.vi" "小时数据发送次数"() -> (w534:i32)
        n296 = Unbundle By Name(w539) -> ("藻密度"=w538:string)
        n297 = Equal?(x=w536, y=w538) -> (x = y?=w526:bool)
        n298 = Index Array(array=w533, index (row)=w534) -> (element=w532:string[])  [unwired: 1 in]
        n299 = Select(t="w00000", s=w526, f=w536) -> (s? t:f=w535:string)
        n300 = Index Array(array=w532, index #1=0 ("索引"), index #2=2 ("索引")) -> (element #1=w523:string, element #2=w545:string)
        n301 = Empty String/Path?(string/path=w545) -> (empty?=w544:bool)
        n302 = Select(t="i22001", s=w526, f="i12001") -> (s? t:f=w525:string)
        n303 = Select(t="i22003", s=w526, f="i12031") -> (s? t:f=w524:string)
        n304 = Number To Decimal String(number=w529) -> (decimal integer string=w530:string)  [unwired: 1 in]
        n305 = Number To Decimal String(number=w513) -> (decimal integer string=w514:string)  [unwired: 1 in]
        n306 = case shown="假" w544 {
          tunnel: [w592 ""] -> w520
          tunnel: w545 -> [w589 _]
          tunnel: w535 -> [w587 _]
          tunnel: w530 -> [w585 _]
          tunnel: w525 -> [w586 _]
          tunnel: w524 -> [w590 _]
          tunnel: w514 -> [w584 _]
          frame False {
            n307 = call "告警信息文本转换为协议i12031值.vi"("字符串"=w589) -> ("十进制整型字符串"=w588:string)  [unwired: 10 in]
            n308 = Format Into String(format string="PolId=%s,%s-Info=%s,i12002-Info=0,i12003-Info=%s,%s-Info=%s;" ("格式字符串"), w587, w586, w585, w584, w590, w588) -> (resulting string=w592:string)  [unwired: 2 in, 1 out]
          }
          frame True {
          }
        }
        n309 = Empty String/Path?(string/path=w520) -> (empty?=w519:bool)
        n310 = Concatenate Strings(w516, w520) -> (w522:string)
        n311 = Not(x=w519) -> (.not. x?=w518:bool)
        n312 = And(x=w515, y=w518) -> (x .and. y?=w517:bool)
        n313 = case shown="真" w517 {
          tunnel: w523 -> [_ w549]
          tunnel: w522 -> [w546 w548]
          tunnel: [w546 w547] -> w521
          frame False {
          }
          frame True {
            n314 = call "规范时间戳.vi"("字符串"=w549) -> ("result string"=w551:string)  [unwired: 10 in]
            n315 = Format Into String(format string="DataTime=%s;%s", w551, w548) -> (resulting string=w547:string)  [unwired: 2 in, 1 out]
          }
        }
      }
    }
  }
  "字符串" <- w19
